vi "ReadSetpointFile-v2.vi"(11 "Setpoint file name":string) -> (0 "Fan Vel Set":dbl[][](array[numeric]), 1 "Rotor Spd Set":dbl[](array[numeric]), 2 "Pitch Set":dbl[](array[numeric]), 3 "Time":dbl[](array[numeric]), 4 "Setpoint file loaded":path, 5 "Setpoint indicator":dbl[][](array[numeric]), 7 "Read error":string)   [LabVIEW 2018]
uses:
  <vilib>/Utility/file.llb/Read Delimited Spreadsheet (DBL).vi
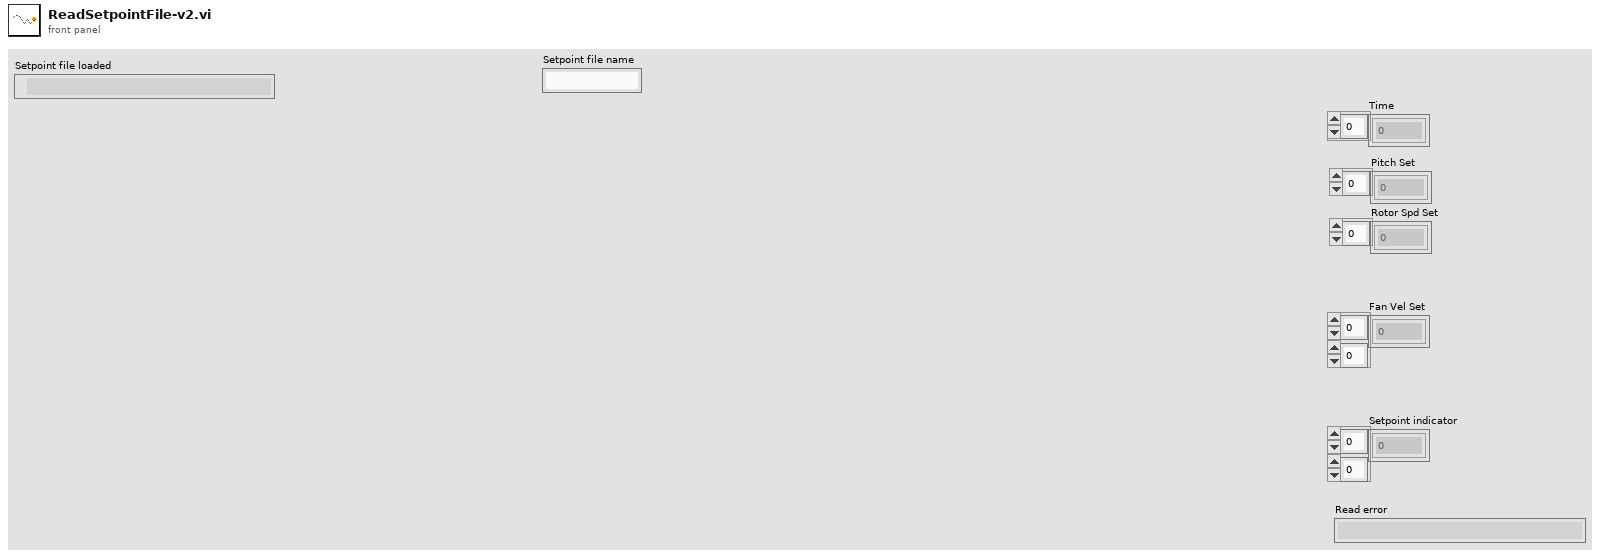
[diagram p1: front panel]
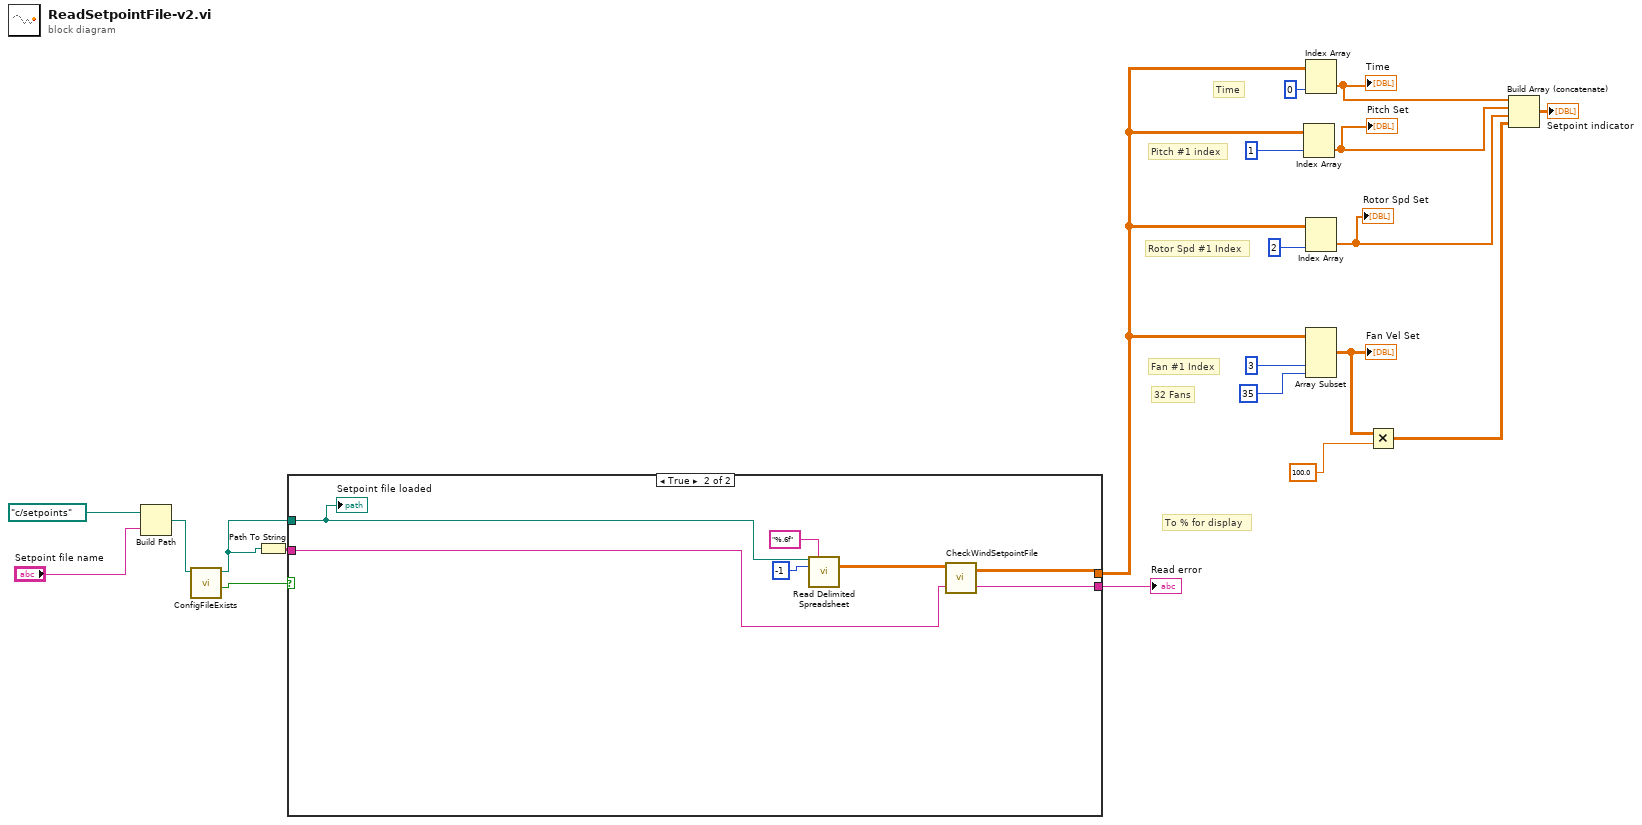
[diagram p0: block diagram]
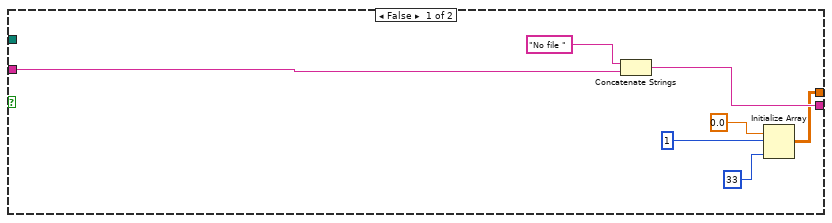
[diagram p2: hidden frame]
diagram:
  # "Rotor Spd #1 Index"
  # "Pitch #1 index"
  # "To % for display"
  # "32 Fans"
  # "Fan #1 Index"
  # "Time"
  n1 = Build Path(base path=path "c:/setpoints" ("file path (dialog if empty)"), name or relative path="Setpoint file name") -> (appended path=w11:path)
  n2 = call "ConfigFileExists.vi"("Path   In"=w11) -> ("file found"=w12:bool, "Path Out"=w10:path)  [unwired: 9 in]
  n3 = Path To String(path=w10) -> (string=w19:string)
  n4 = case shown="True" w12 {
    tunnel: w19 -> [w26 w30]
    tunnel: w10 -> [_ w28]
    tunnel: [w25 w31] -> w18
    tunnel: [w21 w29] -> w3
    frame False {
      n5 = Concatenate Strings("No file ", w26) -> (w25:string)
      n6 = Initialize Array(0.0 ("element"), 1 ("dimension size"), 33 ("dimension size")) -> (w21:dbl[][])
    }
    frame True {
      n7 = call-poly <vilib>:"Read Delimited Spreadsheet.vi"("file path (dialog if empty)"=w28, "format (%.3f)"="%.6f", "number of rows (all:-1)"=-1) -> ("all rows"=w34:dbl[][])  [unwired: 7 in, 5 out]
      n8 = call "CheckWindSetpointFile.vi"("File Name"=w30, "Setpoints In"=w34) -> ("Read error"=w31:string, "Setpoints Out"=w29:dbl[][])
      "Setpoint file loaded" <- w28
    }
  }
  "Read error" <- w18
  n9 = Index Array(array=w3, index (col)=1 ("index")) -> (element=w1:dbl[])  [unwired: 1 in]
  "Pitch Set" <- w1
  n10 = Index Array(array=w3, index (col)=0 ("disabled index (col)")) -> (element=w9:dbl[])  [unwired: 1 in]
  "Time" <- w9
  n11 = Index Array(array=w3, index (col)=2 ("index")) -> (element=w2:dbl[])  [unwired: 1 in]
  "Rotor Spd Set" <- w2
  n12 = Array Subset(array=w3, index (col)=3 ("index"), length (col)=35 ("disabled index (col)")) -> (w8:dbl[][])  [unwired: 2 in]
  "Fan Vel Set" <- w8
  n13 = Multiply(x=w8, y=100.0) -> (x*y=w7:dbl[][])
  n14 = Build Array (concatenate)(w9, w1, w2, w7) -> (→"Setpoint indicator":dbl[][])
